vi "Validate Transmit Mode Codes.vi"(4 "RT Address (0-30)":u8, 6 "RT 1?":bool, 8 "error in (no error)":errorcluster, 11 "1553 Unit Test in":refnum<class "Remote Terminal.lvclass">) -> (0 "error out":errorcluster, 3 "1553 Unit Test out":refnum<class "Remote Terminal.lvclass">)   [LabVIEW 2020, in "Unit Tests.lvlib" / "Remote Terminal.lvclass"]
uses:
  Remote Terminal.lvclass
  Remote Terminal.lvclass/Remote Terminal.ctl
  <vilib>/addons/_JKI Toolkits/Caraya/classes/Assert/Assert True.vi
  Dependencies/FPGA Interface/FPGA Interface.lvclass
  <vilib>/addons/_JKI Toolkits/Caraya/classes/Assert/Assert.lvclass
  <vilib>/addons/_JKI Toolkits/Caraya/classes/Test/Test.lvclass
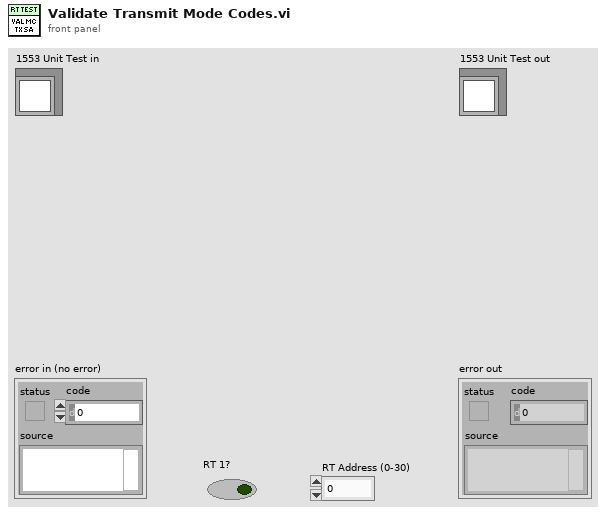
[diagram p1: front panel]
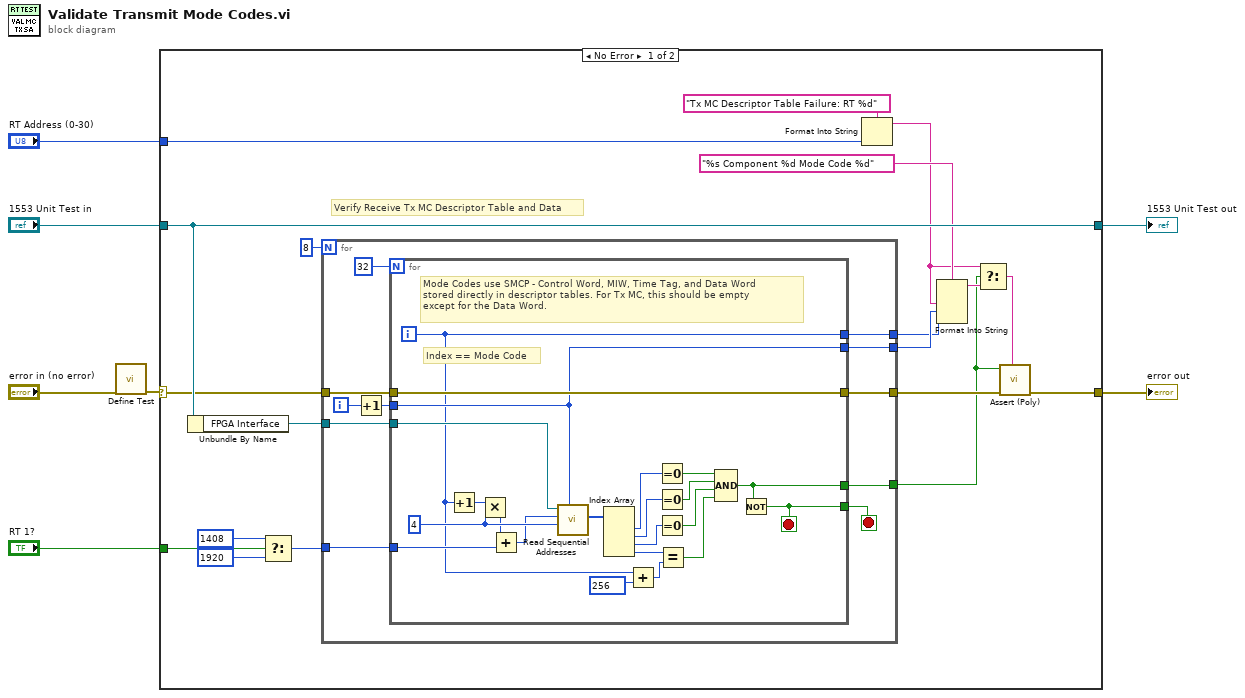
[diagram p0: block diagram]
diagram:
  n1 = call <vilib>:"Define Test.vi"("error in (no error)"="error in (no error)") -> ("error out"=w3:errorcluster)  [unwired: 9 in, 1 out]
  n2 = case shown="No Error" w3 {
    selector: w3 -> [w19 w61]
    tunnel: [w18 w61] -> w7
    tunnel: [w26 w60] -> w5
    tunnel: "1553 Unit Test in" -> [w26 w60]
    tunnel: "RT 1?" -> [w22 _]
    tunnel: "RT Address (0-30)" -> [w13 _]
    frame No Error {
      # "Verify Receive Tx MC Descriptor Table and Data"
      n3 = Unbundle By Name(w26) -> ("FPGA Interface"=w20:refnum<class "FPGA Interface.lvclass">)
      n4 = Select(t=u16 1408, s=w22, f=u16 1920) -> (s? t:f=w21:u16)
      n5 = for {
        N: 8 -> [_]
        tunnel: w21 -> [w29]
        tunnel: w20 -> [w34]
        tunnel: w19 -> [w33]
        tunnel: [w32] -> w9
        tunnel: [w31] -> w11
        tunnel: [w30] -> w10
        tunnel: [w28] -> w8
        i -> [w37]
        stop <- w27 stop-if-true
        n6 = Increment(x=w37) -> (x+1=w35:i32)
        n7 = for {
          N: 32 -> [_]
          tunnel: w35 -> [w57]
          tunnel: w34 -> [w59]
          tunnel: w33 -> [w58]
          tunnel: [w58] -> w32
          tunnel: [w40] -> w28
          tunnel: [w57] -> w31
          tunnel: [w41] -> w30
          tunnel: w29 -> [w53]
          tunnel: [w39] -> w27
          i -> [w41]
          stop <- w39 stop-if-true
          w55 = u16 4 ("x")
          # "Mode Codes use SMCP - Control Word, MIW, Time Tag, and Data Word \nstored directly in descriptor tables. For Tx MC, this should be empty \nexcept for the Data Word."
          # "Index == Mode Code"
          n8 = Increment(x=w41) -> (x+1=w38:i32)
          n9 = Multiply(x=w38, y=w55) -> (x*y=w54:i32)
          n10 = Add(x=w54, y=w53) -> (x+y=w52:i32)
          n11 = call-dynamic "Read Sequential Addresses.vi"("Target IC (1-8)"=w57, "Addresses to Read"=w55, "Starting Address"=w52, "FPGA Interface in"=w59) -> ("Data"=w56:u16[])  [unwired: 6 in, 1 out]
          n12 = Index Array(array=w56) -> (element #1=w51:u16, element #2=w50:u16, element #3=w49:u16, element #4=w44:u16)  [unwired: 4 in]
          n13 = Add(x=w41, y=256) -> (x+y=w43:i32)
          n14 = Equal To 0?(x=w51) -> (x = 0?=w48:bool)
          n15 = Equal To 0?(x=w50) -> (x = 0?=w47:bool)
          n16 = Equal To 0?(x=w49) -> (x = 0?=w46:bool)
          n17 = Equal?(x=w44, y=w43) -> (x = y?=w45:bool)
          n18 = Compound Arithmetic op=AND(w48, w47, w46, w45) -> (w40:bool)
          n19 = Not(x=w40) -> (.not. x?=w39:bool)
        }
      }
      n20 = Format Into String(format string="Tx MC Descriptor Table Failure: RT %d" ("message (\"\")"), w13) -> (resulting string=w12:string)  [unwired: 2 in, 1 out]
      n21 = Format Into String(format string="%s Component %d Mode Code %d" ("message (\"\")"), w12, w11, w10) -> (resulting string=w16:string)  [unwired: 2 in, 1 out]
      n22 = Select(t=w12, s=w8, f=w16) -> (s? t:f=w15:string)
      n23 = call-poly <vilib>:"Assert (Poly).vi"("Label"=w15, "error in (no error)"=w9, "True?"=w8) -> ("error out"=w18:errorcluster)  [unwired: 7 in, 1 out]
    }
    frame Error {
    }
  }
  "error out" <- w7
  "1553 Unit Test out" <- w5
